vi "Debouncing.vi"(9 "Debounce Ticks":u16=5, 11 "Input Signal":bool) -> (3 "Debounced Signal":bool)   [LabVIEW 2015]
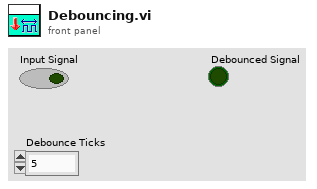
[diagram p1: front panel]
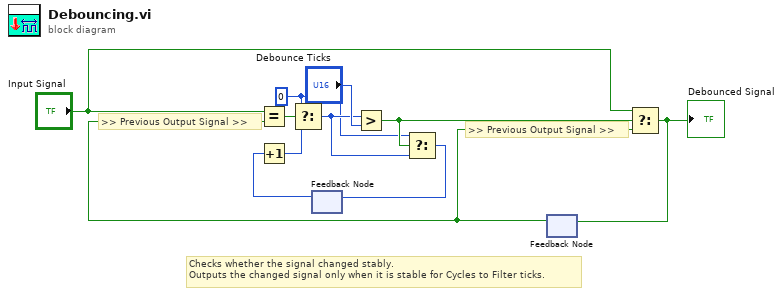
[diagram p0: block diagram]
diagram:
  w1 = u16 0 ("f")
  # "Checks whether the signal changed stably.\nOutputs the changed signal only when it is stable for Cycles to Filter ticks."
  # ">> Previous Output Signal >>"
  # ">> Previous Output Signal >>"
  n1 = feedback #1() -> (w11:u16)  [unwired: 1 out]
  n2 = Increment(x=w11) -> (x+1=w7:u16)
  n3 = feedback #2() -> (w8:bool)  [unwired: 1 out]
  n4 = Equal?(x="Input Signal", y=w8) -> (x = y?=w9:bool)
  n5 = Select(t=w1, s=w9, f=w7) -> (s? t:f=w4:u16)
  n6 = Greater?(x=w4, y="Debounce Ticks") -> (0:w6:bool)
  n7 = Select(t=w1, s=w6, f=w4) -> (s? t:f=w5:u16)
  n8 = feedback-in #1(w5) -> ()
  n9 = Select(t="Input Signal", s=w6, f=w8) -> (s? t:f=w2:bool)
  "Debounced Signal" <- w2
  n10 = feedback-in #2(w2) -> ()
